vi "Check.vi"(8 "error in (no error)":errorcluster, 11 "CEID Data":cluster{"CEID":u32, "RPTID":u32[]}[](array[cluster])) -> (0 "error out":errorcluster, 3 "S2F36":T1)   [LabVIEW 2020, in "SECS Scenarios.lvlib" / "34-CEID Setup.lvclass"]
uses:
  34-CEID Setup.lvclass
  SECS Communication/S2 Message Class/S2F36.ctl
  SECS Communication/SECS Data Class/Get CEID Data.vi
  SECS Communication/SECS Data Class/Get RPTID Data.vi
  SECS Communication/SECS Data Class/Get All CEID Data.vi
  SECS Communication/SECS Data Class/SECS Data Class.lvclass
  SECS Communication/S2 Message Class/S2 Message Class.lvclass
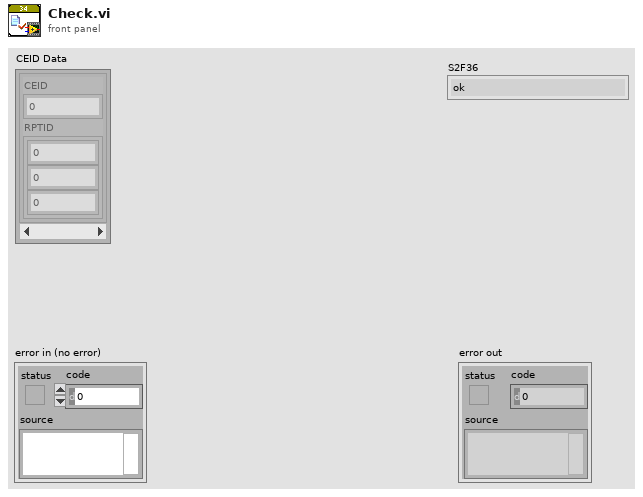
[diagram p1: front panel]
types:
  T1 = typedef "SECS Communication.lvlib/S2 Message Class.lvclass/S2F36.ctl" = enum16{"ok", "out of space", "invalid format", "1 or more CEID links already defined", "1 or more CEID invalid", "1 or more RPTID invalid"}
  T2 = typedef "SECS Communication.lvlib/SECS Data Class.lvclass/CEID Data.ctl" = cluster{"Enable":bool, "CEID":u32, "Name":string, "Description":string, "RPTID":u32[], "Dynamic":bool}
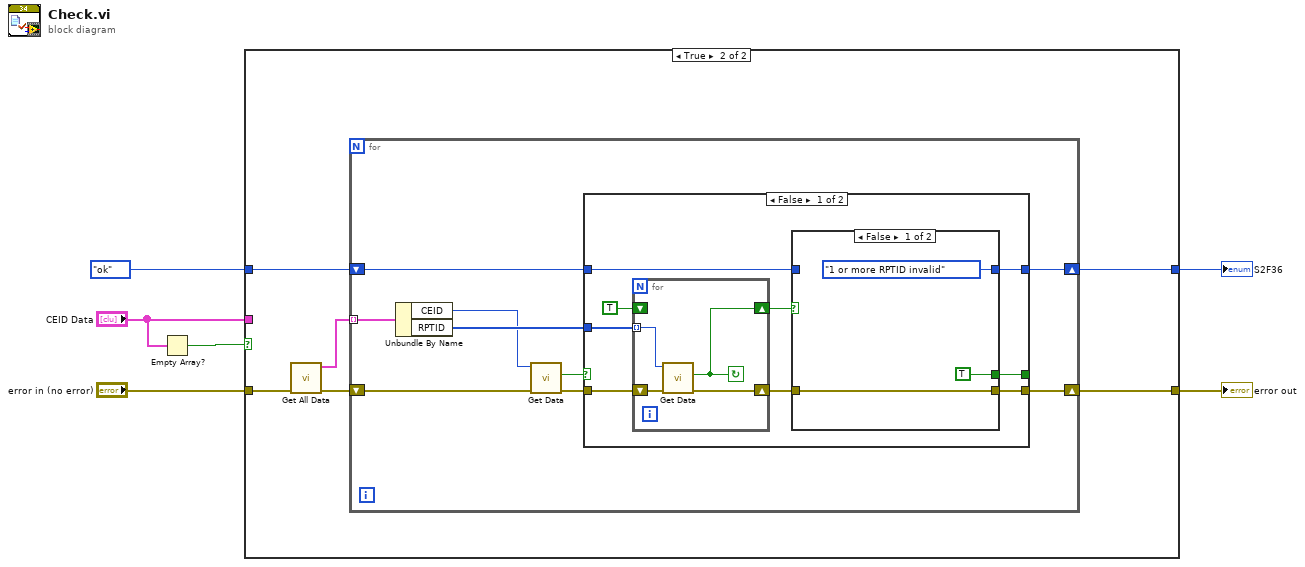
[diagram p0: block diagram]
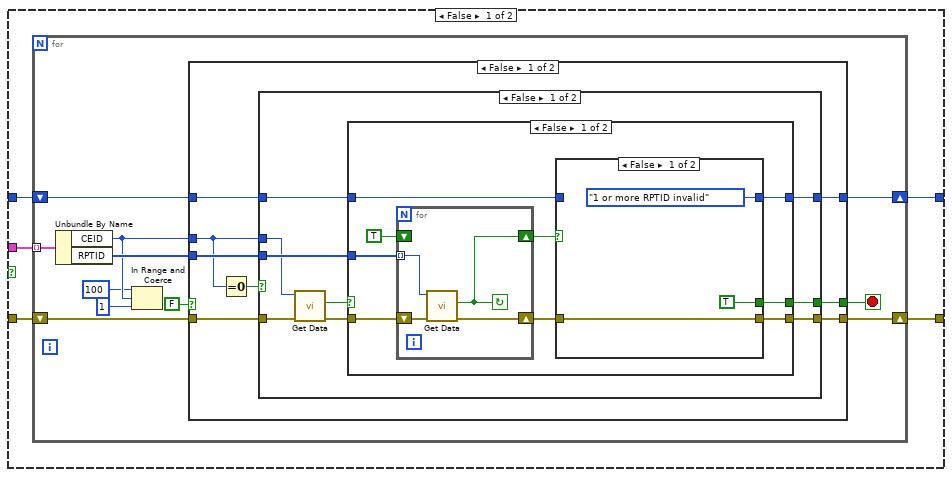
[diagram p2: hidden frame]
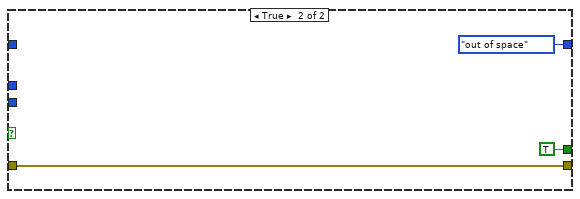
[diagram p5: hidden frame]
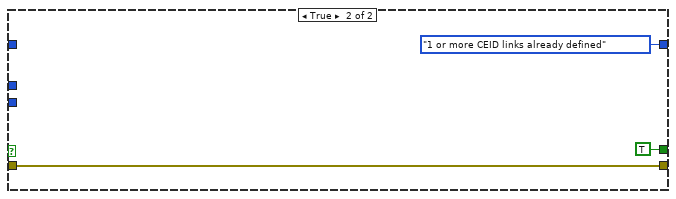
[diagram p6: hidden frame]
diagram:
  n1 = Empty Array?(array="CEID Data") -> (empty?=w1:bool)
  n2 = case shown="True" w1 {
    tunnel: "error in (no error)" -> [w11 w68]
    tunnel: S2F36."ok" ("S2F36") -> [w10 w72]
    tunnel: [w9 w71] -> w4
    tunnel: [w8 w70] -> w3
    tunnel: "CEID Data" -> [w7 _]
    frame False {
      n3 = for {
        tunnel: w7 -> [w22] mode=indexing
        shift-right: [w16] -> w9
        shift-left: w11 -> [w21]
        shift-right: [w17] -> w8
        shift-left: w10 -> [w18]
        stop <- w19 stop-if-true
        n4 = Unbundle By Name(w22) -> ("CEID"=w15:u32, "RPTID"=w20:u32[])
        n5 = In Range and Coerce(upper limit=u32 100, x=w15, lower limit=u32 1) -> ()  [unwired: 2 out]
        n6 = case shown="False" FALSE {
          tunnel: w21 -> [w30 w66]
          tunnel: w20 -> [w29 _]
          tunnel: [w28 TRUE] -> w19
          tunnel: w18 -> [w27 _]
          tunnel: [w26 S2F36."1 or more CEID links already defined" ("S2F36")] -> w17
          tunnel: [w25 w66] -> w16
          tunnel: w15 -> [w24 _]
          frame False {
            n7 = Equal To 0?(x=w24) -> (x = 0?=w23:bool)
            n8 = case shown="False" w23 {
              tunnel: w30 -> [w39 w63]
              tunnel: w29 -> [w36 _]
              tunnel: [w35 TRUE] -> w28
              tunnel: w27 -> [w34 _]
              tunnel: [w33 S2F36."out of space" ("S2F36")] -> w26
              tunnel: [w32 w63] -> w25
              tunnel: w24 -> [w31 _]
              frame False {
                n9 = call-poly "Get Data.vi"("error in"=w39, "CEID"=w31) -> ("error out"=w38:errorcluster, "Find?"=w37:bool)  [unwired: 7 in, 1 out]
                n10 = case shown="False" w37 {
                  selector: w37 -> [_ w59]
                  tunnel: w38 -> [w48 w60]
                  tunnel: w36 -> [w42 _]
                  tunnel: [w43 w59] -> w35
                  tunnel: [w44 w60] -> w32
                  tunnel: w34 -> [w46 w58]
                  tunnel: [w45 w58] -> w33
                  frame False {
                    n11 = for {
                      shift-right: [w55] -> w47
                      shift-left: w48 -> [w57]
                      tunnel: w42 -> [w56] mode=indexing
                      shift-right: [w54] -> w40
                      shift-left: TRUE -> [_]
                      stop <- w54 continue-if-true
                      n12 = call-poly "Get Data.vi"("error in"=w57, "RPTID"=w56) -> ("error out"=w55:errorcluster, "Find?"=w54:bool)  [unwired: 7 in, 1 out]
                    }
                    n13 = case shown="False" w40 {
                      tunnel: w47 -> [w51 w52]
                      tunnel: w46 -> [_ w53]
                      tunnel: [S2F36."1 or more RPTID invalid" ("S2F36") w53] -> w45
                      tunnel: [w51 w52] -> w44
                      tunnel: [TRUE _] -> w43
                      frame False {
                      }
                      frame True {
                      }
                    }
                  }
                  frame True {
                  }
                }
              }
              frame True {
              }
            }
          }
          frame True {
          }
        }
      }
    }
    frame True {
      n14 = call-poly "Get All Data.vi"("error in (no error)"=w68) -> ("error out"=w67:errorcluster, "CEID Data"=w69:T2[])  [unwired: 9 in]
      n15 = for {
        shift-right: [w79] -> w71
        shift-left: w67 -> [w81]
        shift-right: [w78] -> w70
        shift-left: w72 -> [w80]
        tunnel: w69 -> [w73] mode=indexing
        n16 = Unbundle By Name(w73) -> ("CEID"=w76:u32, "RPTID"=w77:u32[])
        n17 = call-poly "Get Data.vi"("error in"=w81, "CEID"=w76) -> ("error out"=w75:errorcluster, "Find?"=w74:bool)  [unwired: 7 in, 1 out]
        n18 = case shown="False" w74 {
          selector: w74 -> [_ w101]
          tunnel: w75 -> [w90 w102]
          tunnel: w77 -> [w84 _]
          tunnel: [w85 w101] -> _
          tunnel: [w86 w102] -> w79
          tunnel: w80 -> [w88 w100]
          tunnel: [w87 w100] -> w78
          frame False {
            n19 = for {
              shift-right: [w97] -> w89
              shift-left: w90 -> [w99]
              tunnel: w84 -> [w98] mode=indexing
              shift-right: [w96] -> w82
              shift-left: TRUE -> [_]
              stop <- w96 continue-if-true
              n20 = call-poly "Get Data.vi"("error in"=w99, "RPTID"=w98) -> ("error out"=w97:errorcluster, "Find?"=w96:bool)  [unwired: 7 in, 1 out]
            }
            n21 = case shown="False" w82 {
              tunnel: w89 -> [w93 w94]
              tunnel: w88 -> [_ w95]
              tunnel: [S2F36."1 or more RPTID invalid" ("S2F36") w95] -> w87
              tunnel: [w93 w94] -> w86
              tunnel: [TRUE _] -> w85
              frame False {
              }
              frame True {
              }
            }
          }
          frame True {
          }
        }
      }
    }
  }
  "error out" <- w4
  "S2F36" <- w3
